vi "Set Motor On_OFF.vi"(8 "error in (no error)":errorcluster, 10 "ON/OFF":bool, 11 "FujiMotor in":refnum<class "FujiMotor.lvclass">) -> (0 "error out":errorcluster, 3 "FujiMotor out":refnum<class "FujiMotor.lvclass">)   [LabVIEW 2014, in "ALPHA5 RS485.lvlib" / "FujiMotor.lvclass"]
uses:
  FujiMotor.lvclass
  FujiMotor.lvclass/FujiMotor.ctl
  ALPHA5 RS485.lvlib
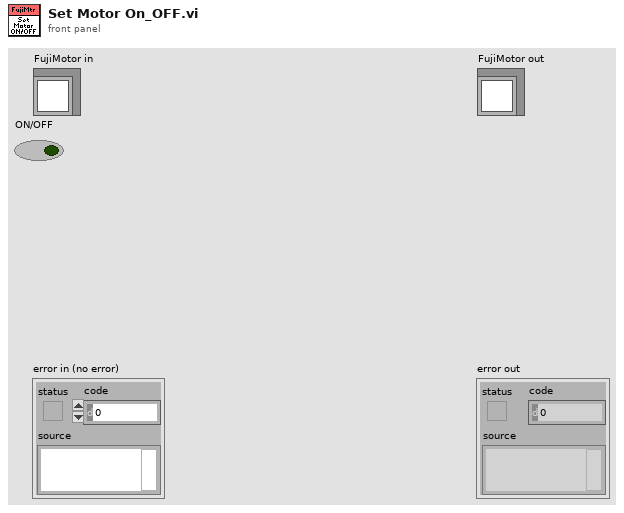
[diagram p1: front panel]
types:
  T1 = typedef "ALPHA5 RS485.lvlib/Port Selection Info.ctl" = cluster{"Port Name":refnum<visa-resource-name>, "Amplifier Num":u8, "Baud Rate":u32, "Char Formation":enum16{"0", "1", "2", "3", "4", "5"}}
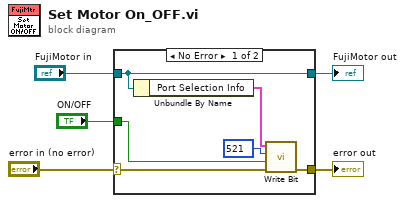
[diagram p0: block diagram]
diagram:
  n1 = case shown="No Error" "error in (no error)" {
    selector: "error in (no error)" -> [w9 w12]
    tunnel: [w8 w12] -> w4
    tunnel: [w11 w13] -> w2
    tunnel: "FujiMotor in" -> [w11 w13]
    tunnel: "ON/OFF" -> [w6 _]
    frame No Error {
      n2 = Unbundle By Name(w11) -> ("Port Selection Info"=w10:T1)
      n3 = call "Write Bit.vi"("error in (no error)"=w9, "ON/OFF"=w6, "Address"=u16 521, "Port Selection Info In"=w10) -> ("error out"=w8:errorcluster)  [unwired: 6 in, 1 out]
    }
    frame Error {
    }
  }
  "error out" <- w4
  "FujiMotor out" <- w2
